vi "DoAttack.vi"(8 "error in (no error)":errorcluster, 10 "Rival":refnum<class "Peasant.lvclass">, 11 "Accessory in":refnum<class "Accessory.lvclass">) -> (0 "error out":errorcluster, 2 "Rival":refnum<class "Peasant.lvclass">, 3 "Accessory out":refnum<class "Accessory.lvclass">)   [LabVIEW 2021, in "Accessory.lvclass"]
uses:
  Accessory.lvclass
  Peasant/Peasant.lvclass
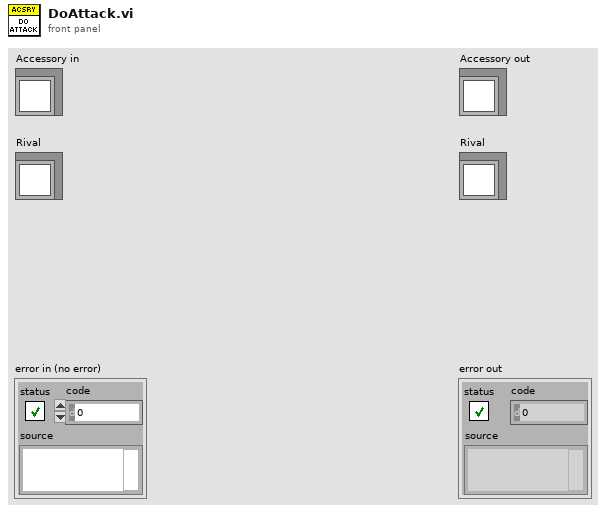
[diagram p1: front panel]
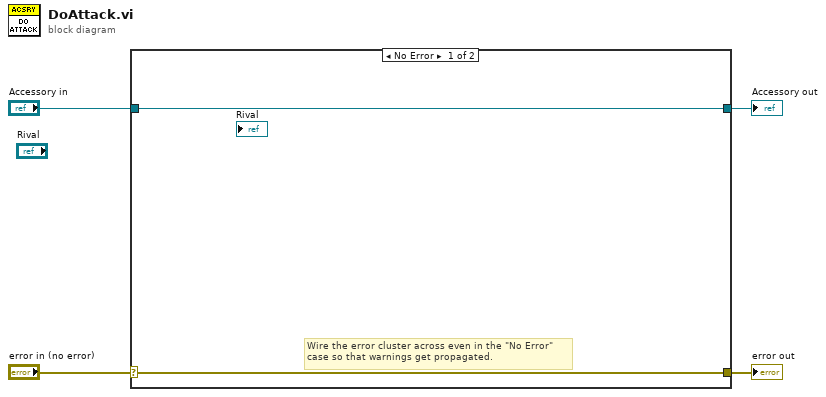
[diagram p0: block diagram]
diagram:
  n1 = case shown="No Error" "error in (no error)" {
    selector: "error in (no error)" -> [w5 w8]
    tunnel: [w5 w8] -> w3
    tunnel: [w6 w7] -> w1
    tunnel: "Accessory in" -> [w6 w7]
    frame No Error {
      # "Wire the error cluster across even in the \"No Error\"\ncase so that warnings get propagated."
    }
    frame Error {
    }
  }
  "error out" <- w3
  "Accessory out" <- w1
